vi "dc.vi"(2 "c":bool, 3 "d":bool) -> (0 "not q":bool, 1 "q":bool)   [LabVIEW 2012]
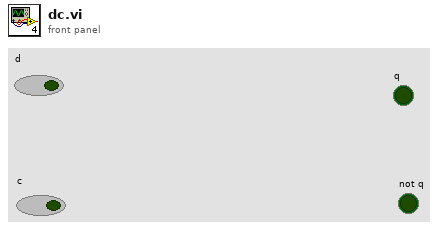
[diagram p1: front panel]
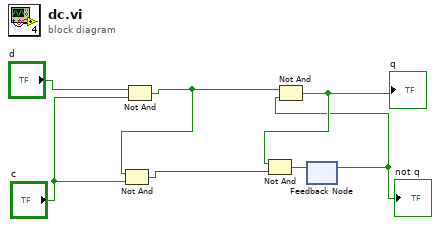
[diagram p0: block diagram]
diagram:
  n1 = Not And(1:"c", 2:"d") -> (0:w5:bool)
  n2 = Not And(1:"c", 2:w5) -> (0:w4:bool)
  n3 = feedback #1() -> (w1:bool)  [unwired: 1 in]
  "not q" <- w1
  n4 = Not And(1:w1, 2:w5) -> (0:w3:bool)
  "q" <- w3
  n5 = Not And(1:w4, 2:w3) -> (0:w2:bool)
  n6 = feedback-in #1(w2) -> ()
